vi "Oracle Popup.vi"(8 "error in":errorcluster, 10 "Calling VI Refnum in":refnum<vi>, 11 "SR List in":T1[](array[typedef]) {"Creation Date" format="%<%x>T"; "Last Updated" format="%<%x>T"}) -> (0 "error out":errorcluster, 3 "SR List out":T1[](array[typedef]) {"Creation Date" format="%<%x>T"; "Last Updated" format="%<%x>T"})   [LabVIEW 2018]
uses:
  <vilib>/Utility/miscctls.llb/LVPointTypeDef.ctl
  Type Defs/SR Cluster.ctl
  Type Defs/SR Status.ctl
panel:
  in  "Ok Button":bool
  in  "Copied Text":string
  in  "Close":bool
  # "In your Universal Work Queue in Oracle, right-click anywhere in the table and select \"Copy All Rows.\" Paste the copied information in the string container below, then press \"OK\"."
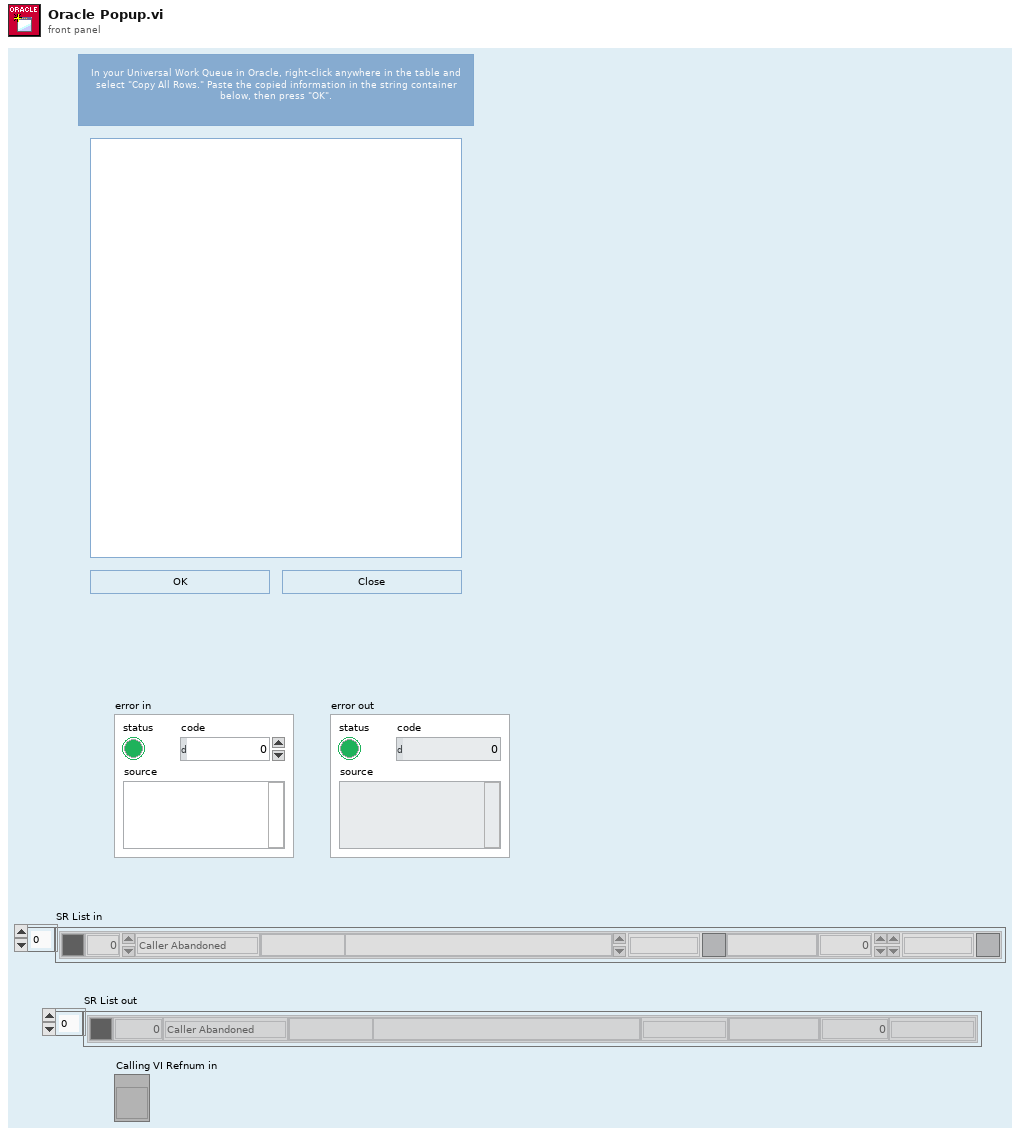
[diagram p1: front panel]
types:
  T1 = typedef "SR Cluster.ctl" = cluster{"Color":u32, "SR Number":i32, "SR Status":T2, "SR Type":string, "Summary":string, "Last Updated":timestamp, "Service Level":string, "Days Open":dbl, "Creation Date":timestamp}
  T2 = typedef "SR Status.ctl" = enum16{"Caller Abandoned", "Created in Error", "Expired", "Forum Resolved AE", "Forum Resolved Customer", "IN WORK", "IN WORK Collab with AES", "IN WORK Collab with PSE", "IN WORK Collab with SE", "IN WORK Customer Added Note", "IN WORK Escalation", "IN WORK Wait on Customer", "Open", "Potentially Resolved", "Presumed Resolved", "RMA Approved for Return", "Resolved", "Passed Off"}
  T3 = typedef "LVPointTypeDef.ctl" = cluster{"Horizontal":i16, "Vertical":i16}
  T4 = typedef "LVRectTypeDef.ctl" = cluster{"Left":i16, "Top":i16, "Right":i16, "Bottom":i16}
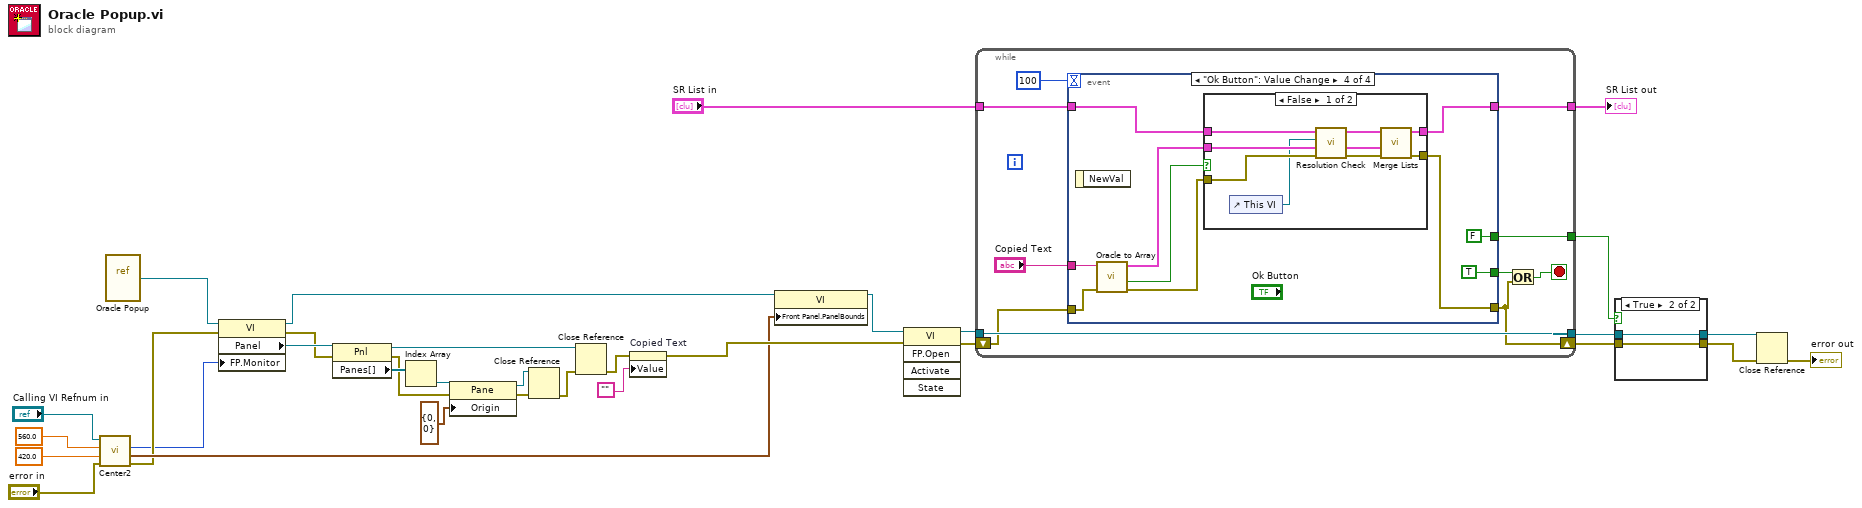
[diagram p0: block diagram]
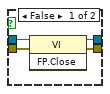
[diagram p2: hidden frame]
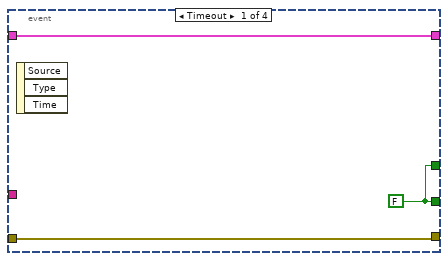
[diagram p3: hidden frame]
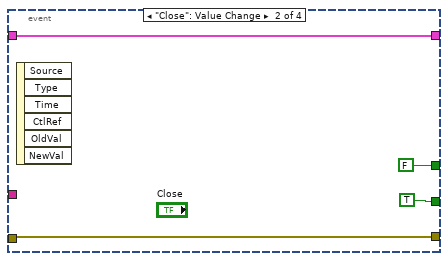
[diagram p4: hidden frame]
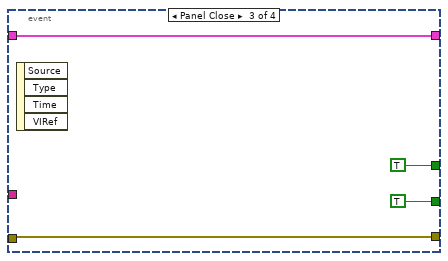
[diagram p5: hidden frame]
diagram:
  n1 = call "Center2.vi"("error in (no error)"="error in", "Width"=420.0, "Height"=560.0, "VI in"="Calling VI Refnum in") -> ("error out"=w5:errorcluster, "New Bounds"=w6:T4, "Active Monitor"=w1:u16)  [unwired: 5 in]
  n2 = vi-ref "Oracle Popup.vi"() -> (w29:refnum<vi>)
  n3 = property class="VI"(reference=w29, error in=w5, "FP.Monitor"=w1) -> (reference out=w8:refnum<vi>, error out=w19:errorcluster, "Panel"=w20:refnum<vi>)
  n4 = property class="Pnl"(reference=w20, error in=w19) -> (reference out=w21:refnum<vi>, error out=w26:errorcluster, "Panes[]"=w28:refnum<vi>[])
  n5 = Index Array(array=w28) -> (element=w27:refnum<vi>)  [unwired: 1 in]
  n6 = property class="Pane"(reference=w27, error in=w26, "Origin"=T3 {"Horizontal"=0, "Vertical"=0}) -> (reference out=w24:refnum<vi>, error out=w23:errorcluster)
  n7 = Close Reference(reference=w24, error in (no error)=w23) -> (error out=w22:errorcluster)
  n8 = Close Reference(reference=w21, error in (no error)=w22) -> (error out=w11:errorcluster)
  n9 = property on="Copied Text" class="Str"(error in=w11, "Value"="") -> (error out=w9:errorcluster)  [unwired: 1 in, 1 out]
  n10 = property class="VI"(reference=w8, "Front Panel.PanelBounds"=w6) -> (reference out=w7:refnum<vi>)  [unwired: 1 in, 1 out]
  n11 = invoke class="VI" method="FP.Open"(reference=w7, error in=w9) -> (reference out=w13:refnum<vi>, error out=w12:errorcluster)  [unwired: 3 in, 3 out]
  n12 = while {
    tunnel: [w43] -> w33
    tunnel: w13 -> [w43]
    tunnel: [w41] -> w18
    tunnel: "SR List in" -> [w40]
    shift-right: [w35] -> w32
    shift-left: w12 -> [w38]
    tunnel: [w34] -> w14
    stop <- w36 stop-if-true
    n13 = event shown="[3] \"Ok Button\": Value Change" {
      selector: _ -> [_ _ _ _]
      dyn-events: _ -> [_ _ _ _]
      timeout: 100 -> [_ _ _ _]
      tunnel: [w44 TRUE ("Stop") TRUE ("Stop") TRUE ("Stop")] -> w37
      tunnel: [w46 w49 w54 w59] -> w41
      tunnel: w40 -> [w46 w49 w54 w60]
      tunnel: "Copied Text" -> [_ _ _ w63]
      tunnel: w38 -> [w45 w48 w52 w62]
      tunnel: [w45 w48 w52 w57] -> w35
      tunnel: [w44 FALSE ("Stop") TRUE ("Stop") FALSE ("Stop")] -> w34
      event Timeout {
        w44 = FALSE ("Stop")
        n14 = event-data() -> ()  [unwired: 1 in, 3 out]
      }
      event "Close": Value Change {
        n15 = event-data() -> ()  [unwired: 1 in, 6 out]
      }
      event Panel Close {
        n16 = event-data() -> ()  [unwired: 1 in, 4 out]
      }
      event "Ok Button": Value Change {
        n17 = event-data() -> ()  [unwired: 1 in, 1 out]
        n18 = call "Oracle to Array.vi"("error in"=w62, "string in"=w63) -> ("error out"=w56:errorcluster, "Empty?"=w61:bool, "list out"=w58:T1[])  [unwired: 7 in]
        n19 = case shown="False" w61 {
          tunnel: w60 -> [w73 w75]
          tunnel: [w70 w75] -> w59
          tunnel: w58 -> [w72 _]
          tunnel: [w68 w74] -> w57
          tunnel: w56 -> [w71 w74]
          frame False {
            n20 = control-ref of="This VI"() -> (w65:refnum<vi>)
            n21 = call "Resolution Check.vi"("error in"=w71, "new list in"=w72, "VI in"=w65, "SR List in"=w73) -> ("error out"=w67:errorcluster, "new list out"=w66:T1[], "list out"=w69:T1[])  [unwired: 5 in]
            n22 = call "Merge Lists.vi"("error in"=w67, "new list in"=w66, "list in"=w69) -> ("error out"=w68:errorcluster, "list out"=w70:T1[])  [unwired: 7 in]
          }
          frame True {
          }
        }
      }
    }
    n23 = Or(x=w37, y=w35) -> (x .or. y?=w36:bool)
  }
  "SR List out" <- w18
  n24 = case shown="True" w14 {
    tunnel: w33 -> [w79 w81]
    tunnel: w32 -> [w78 w80]
    tunnel: [w77 w81] -> w31
    tunnel: [w76 w80] -> w30
    frame False {
      n25 = invoke class="VI" method="FP.Close"(reference=w79, error in=w78) -> (reference out=w77:refnum<vi>, error out=w76:errorcluster)  [unwired: 1 in, 1 out]
    }
    frame True {
    }
  }
  n26 = Close Reference(reference=w31, error in (no error)=w30) -> (error out=→"error out":errorcluster)
